vi "niDAQmx Get Task Property (Name).vi"(0 "task in":refnum<class "Session Factory.lvclass">, 11 "error in":errorcluster) -> (4 "task out":refnum<class "Session Factory.lvclass">, 6 "Name":refnum<k21>, 15 "error out":errorcluster)   [LabVIEW 2021, in "Session Management niDAQmx.lvlib" / "Session Factory.lvclass"]
doc: "<B>Property: Get DAQmx Task (Name)</B>\n\nIndicates the name of the task."
uses:
  Session Factory.lvclass
  Session Factory.lvclass/Session Factory.ctl
  NI DAQmx Client/RPC Messages/nidevice_grpc_Session.ctl
  NI DAQmx Client/NI_DAQmx_client.lvlib
  NI DAQmx Client/RPC Messages/nidaqmx_grpc_GetTaskAttributeStringRequest.ctl
  NI DAQmx Client/RPC Messages/nidaqmx_grpc_TaskStringAttribute.ctl
  NI DAQmx Client/RPC Messages/nidaqmx_grpc_GetTaskAttributeStringRequest_attribute_enum/nidaqmx_grpc_GetTaskAttributeStringRequest_attribute_enum.lvclass
  NI DAQmx Client/RPC Messages/nidevice_grpc_Session_session/nidevice_grpc_Session_session.lvclass
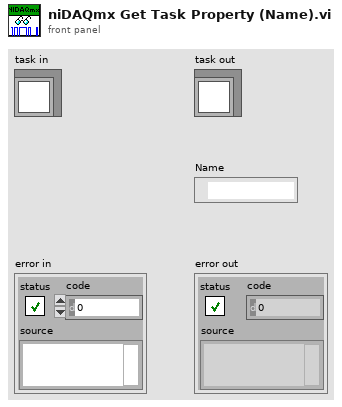
[diagram p1: front panel]
types:
  T1 = typedef "NI_DAQmx_client.lvlib/nidaqmx_grpc_TaskStringAttribute.ctl" = enum32{"TASK_STRING_ATTRIBUTE_UNSPECIFIED", "TASK_ATTRIBUTE_CHANNELS", "TASK_ATTRIBUTE_NAME", "TASK_ATTRIBUTE_DEVICES"}
  T2 = typedef "NI_DAQmx_client.lvlib/nidaqmx_grpc_GetTaskAttributeStringRequest.ctl" = cluster{"task":T3, "nidaqmx_grpc_GetTaskAttributeStringRequest_attribute_enum":refnum<class "nidaqmx_grpc_GetTaskAttributeStringRequest_attribute_enum.lvclass">}
  T3 = typedef "NI_DAQmx_client.lvlib/nidevice_grpc_Session.ctl" = cluster{"nidevice_grpc_Session_session":refnum<class "nidevice_grpc_Session_session.lvclass">}
  T4 = typedef "grpc-lvsupport-release.lvlib/grpcId.ctl" = u64
  T5 = typedef "NI_DAQmx_client.lvlib/nidaqmx_grpc_GetTaskAttributeStringResponse.ctl" = cluster{"status":i32, "value":string}
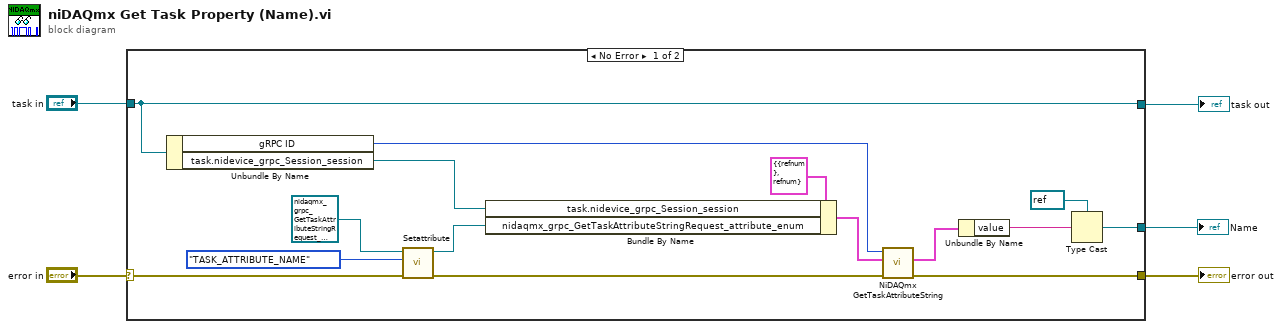
[diagram p0: block diagram]
diagram:
  n1 = case shown="No Error" "error in" {
    selector: "error in" -> [w15 w22]
    tunnel: [w11 w22] -> w4
    tunnel: "task in" -> [w10 w21]
    tunnel: [w10 w21] -> w2
    tunnel: [w7 _] -> w1
    frame No Error {
      n2 = Unbundle By Name(w10) -> ("gRPC ID"=w17:T4, "task.nidevice_grpc_Session_session"=w20:refnum<class "nidevice_grpc_Session_session.lvclass">)
      n3 = call "Setattribute.vi"("error in (no error)"=w15, "Set_Val"=nidaqmx_grpc_TaskStringAttribute."TASK_ATTRIBUTE_NAME", "OneOfTemplate in"=refnum<class "nidaqmx_grpc_GetTaskAttributeStringRequest_attribute_enum.lvclass"> refnum) -> ("error out"=w14:errorcluster, "OneOfTemplate out"=w13:refnum<class "nidaqmx_grpc_GetTaskAttributeStringRequest_attribute_enum.lvclass">)  [unwired: 7 in]
      n4 = Bundle By Name(cluster=T2 {"task"={"nidevice_grpc_Session_session"=refnum}, "nidaqmx_grpc_GetTaskAttributeStringRequest_attribute_enum"=refnum} ("Request Data"), "task.nidevice_grpc_Session_session"=w20, "nidaqmx_grpc_GetTaskAttributeStringRequest_attribute_enum"=w13) -> (w18:T2)
      n5 = call "NiDAQmx GetTaskAttributeString.vi"("error in"=w14, "Request Data"=w18, "gRPC ID"=w17) -> ("error out"=w11:errorcluster, "Response Data"=w16:T5)  [unwired: 6 in, 1 out]
      n6 = Unbundle By Name(w16) -> ("value"=w9:string)
      n7 = Type Cast(type=refnum<k21> refnum ("Name"), x=w9) -> (*(type *) &x=w7:refnum<k21>)
    }
    frame Error {
    }
  }
  "error out" <- w4
  "task out" <- w2
  "Name" <- w1
